vi "Configure Unguided Calibration.vi"(7 "Calibration Method (0: None)":i32(ring) items=["None", "Response Open", "Response Short", "Full 1 Port", "Response", "Receiver Power Cal", "Response Thru", "Response Thru & Isol", "Full SOLT 2 Port", "Full SOLT 3 port", "TRL Call"], 8 "error in (no error)":errorcluster, 9 "Calibration Kit (1)":i32=1, 10 "Channel (1)":i32=1, 11 "VISA resource name":refnum<visa-resource-name>) -> (0 "error out":errorcluster, 3 "VISA resource name out":refnum<visa-resource-name>)   [LabVIEW 2018, in "Keysight PNA Series.lvlib"]
doc: "Configures the Cal Kit and the calibration method for UNGUIDED calibration."
uses:
  Keysight PNA Series.lvlib
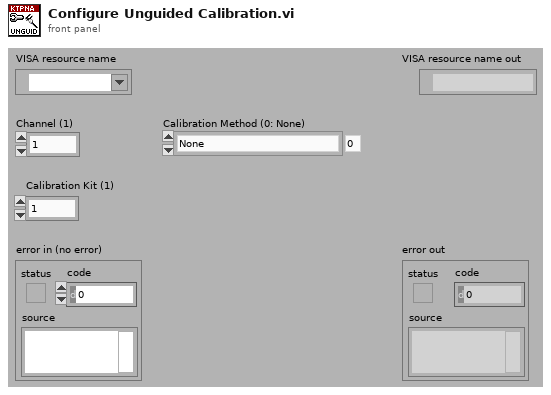
[diagram p1: front panel]
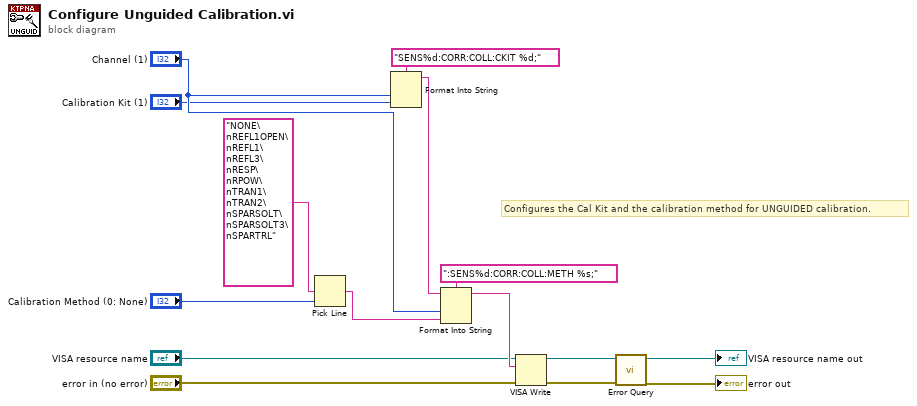
[diagram p0: block diagram]
diagram:
  # "Configures the Cal Kit and the calibration method for UNGUIDED calibration."
  n1 = Pick Line(multi-line string="NONE\nREFL1OPEN\nREFL1\nREFL3\nRESP\nRPOW\nTRAN1\nTRAN2\nSPARSOLT\nSPARSOLT3\nSPARTRL", line index="Calibration Method (0: None)") -> (output string=w8:string)  [unwired: 1 in]
  n2 = Format Into String(format string="SENS%d:CORR:COLL:CKIT %d;", "Channel (1)", "Calibration Kit (1)") -> (resulting string=w10:string)  [unwired: 2 in, 1 out]
  n3 = Format Into String(format string=":SENS%d:CORR:COLL:METH %s;", initial string=w10, "Channel (1)", w8) -> (resulting string=w7:string)  [unwired: 1 in, 1 out]
  n4 = VISA Write(VISA resource name="VISA resource name", write buffer=w7, error in (no error)="error in (no error)") -> (VISA resource name out=w4:refnum<visa-resource-name>, error out=w3:errorcluster)  [unwired: 1 out]
  n5 = call "Error Query.vi"("error in (no error)"=w3, "VISA resource name"=w4) -> ("error out"=→"error out":errorcluster, "VISA resource name out"=→"VISA resource name out":refnum<visa-resource-name>)  [unwired: 6 in, 2 out]
